vi "GetStatus.vi"(1 "connection ID in":refnum<k5>, 3 "error in":errorcluster) -> (7 "InterlLoc State":bool, 8 "OutState":bool, 9 "Fault":bool, 11 "Rem|Loc":bool, 15 "connection ID out":refnum<k5>, 17 "error out":errorcluster)   [LabVIEW 2013]
uses:
  <vilib>/regexp/Match Regular Expression.xnode
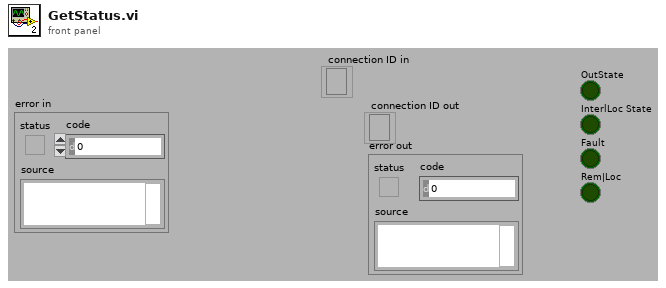
[diagram p1: front panel]
types:
  T1 = enum16{"Standard", "Buffered", "CRLF", "Immediate"}
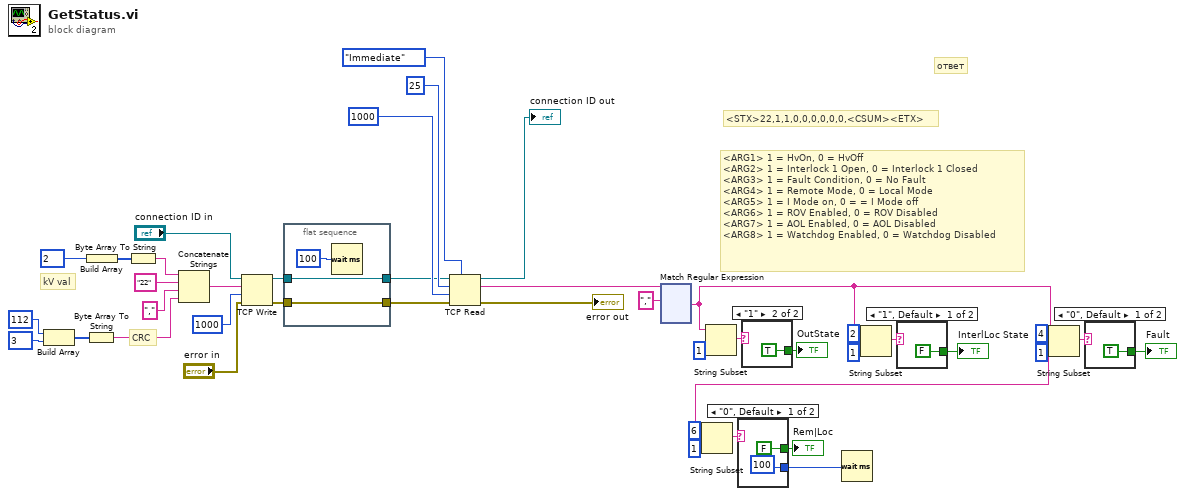
[diagram p0: block diagram]
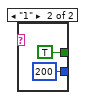
[diagram p2: hidden frame]
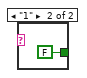
[diagram p3: hidden frame]
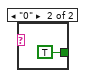
[diagram p4: hidden frame]
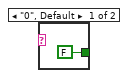
[diagram p5: hidden frame]
diagram:
  # "ответ"
  # "<ARG1> 1 = HvOn, 0 = HvOff\n<ARG2> 1 = Interlock 1 Open, 0 = Interlock 1 Closed\n<ARG3> 1 = Fault Condition, 0 = No Fault\n<ARG4> 1 = Remote Mode, 0 = Local Mode\n<ARG5> 1 = I Mode on, 0 = = I Mode off\n<ARG6> 1 = ROV Enabled, 0 = ROV Disabled\n<ARG7> 1 = AOL Enabled, 0 = AOL Disabled\n<ARG8> 1 = Watchdog Enabled, 0 = Watchdog Disabled"
  # "<STX>22,1,1,0,0,0,0,0,0,<CSUM><ETX>"
  # "CRC"
  # "kV val"
  n1 = Build Array(u8 112 ("y"), u8 3 ("y")) -> (w38:u8[])
  n2 = Byte Array To String(unsigned byte array=w38) -> (string=w29:string)
  n3 = Build Array(u8 2 ("y")) -> (w36:u8[])
  n4 = Byte Array To String(unsigned byte array=w36) -> (string=w35:string)
  n5 = Concatenate Strings(w35, "22" ("string"), "," ("string"), w29) -> (w32:string)
  n6 = TCP Write(connection ID="connection ID in", data in=w32, error in (no error)="error in", 9:1000 ("timeout ms (25000)")) -> (connection ID out=w23:refnum<k5>, error out=w25:errorcluster)  [unwired: 1 out]
  n7 = flat-sequence {
    tunnel: w25 -> [w44]
    tunnel: [w44] -> w24
    tunnel: [w42] -> w22
    tunnel: w23 -> [w42]
    frame #0 {
      n8 = Wait (ms)(milliseconds to wait=u32 100 ("millisecond multiple")) -> ()  [unwired: 1 out]
    }
  }
  n9 = TCP Read(connection ID=w22, bytes to read=25, error in (no error)=w24, 7:T1."Immediate" ("mode (standard)"), 9:1000 ("timeout ms (25000)")) -> (connection ID out=→"connection ID out":refnum<k5>, data out=w2:string, error out=→"error out":errorcluster)
  n10 = xnode "Match Regular Expression"("input string"=w2, "regular expression"=",") -> ("after match"=w4:string)  [unwired: 4 in, 4 out]
  n11 = String Subset(string=w4, offset (0)=6, length (rest)=1 ("length (rest)")) -> (substring=w6:string)
  n12 = String Subset(string=w4, length (rest)=1 ("length (rest)")) -> (substring=w17:string)  [unwired: 1 in]
  n13 = case shown="\"0\", Default" w6 {
    tunnel: [FALSE TRUE] -> w7
    tunnel: [u32 100 ("milliseconds to wait") u32 200 ("milliseconds to wait")] -> w1
    frame "0", Default {
    }
    frame "1" {
    }
  }
  "Rem|Loc" <- w7
  n14 = case shown="\"1\"" w17 {
    tunnel: [FALSE TRUE] -> w16
    frame "0", Default {
    }
    frame "1" {
    }
  }
  "OutState" <- w16
  n15 = Wait (ms)(milliseconds to wait=w1) -> ()  [unwired: 1 out]
  n16 = String Subset(string=w4, offset (0)=2, length (rest)=1 ("length (rest)")) -> (substring=w14:string)
  n17 = case shown="\"1\", Default" w14 {
    tunnel: [FALSE TRUE] -> w15
    frame "1", Default {
    }
    frame "0" {
    }
  }
  "InterlLoc State" <- w15
  n18 = String Subset(string=w4, offset (0)=4, length (rest)=1 ("length (rest)")) -> (substring=w11:string)
  n19 = case shown="\"0\", Default" w11 {
    tunnel: [TRUE FALSE] -> w10
    frame "0", Default {
    }
    frame "1" {
    }
  }
  "Fault" <- w10
